vi "SetNag_report.vi"() -> ()   [LabVIEW 2013]
panel:
  out "Read 14":string
  in  "Write 13":string
  out "Read 13":string
  in  "Write 12":string
  out "Read 12":string
  in  "Write 11":string
  out "Read 11":string
  in  "Write 10":string
  in  "Write 9":string
  out "Read 10":string
  out "Read 9":string
  in  "Write 8":string
  in  "Write 7":string
  out "Read 8":string
  out "Read 7":string
  in  "Write 6":string
  out "Read 6":string
  in  "Write 5":string
  in  "milliseconds to wait":u32=250
  out "Read 5":string
  in  "Write 4":string
  out "Read 3":string
  in  "Baud Rate 2":i32(ring)=2 items=["2400", "4800", "9600", "19200", "38400", "57600", "115200"]
  in  "Com Port 2":i32(ring) items=["Com 1", "Com 2", "Com 3", "Com 4", "Com 5", "Com 6", "COM 7", "COM 8", "COM 9", "COM 10", "COM 11", "COM 12", "com 13", "COM 14"]
  in  "Write 3":string
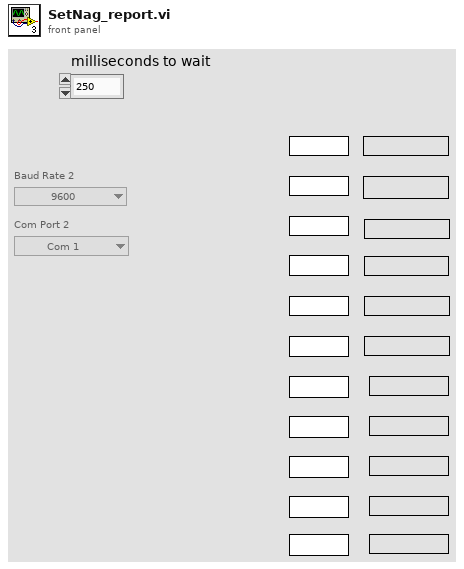
[diagram p1: front panel]
types:
  T1 = enum16{"no parity", "odd parity", "even parity", "mark parity", "space parity"}
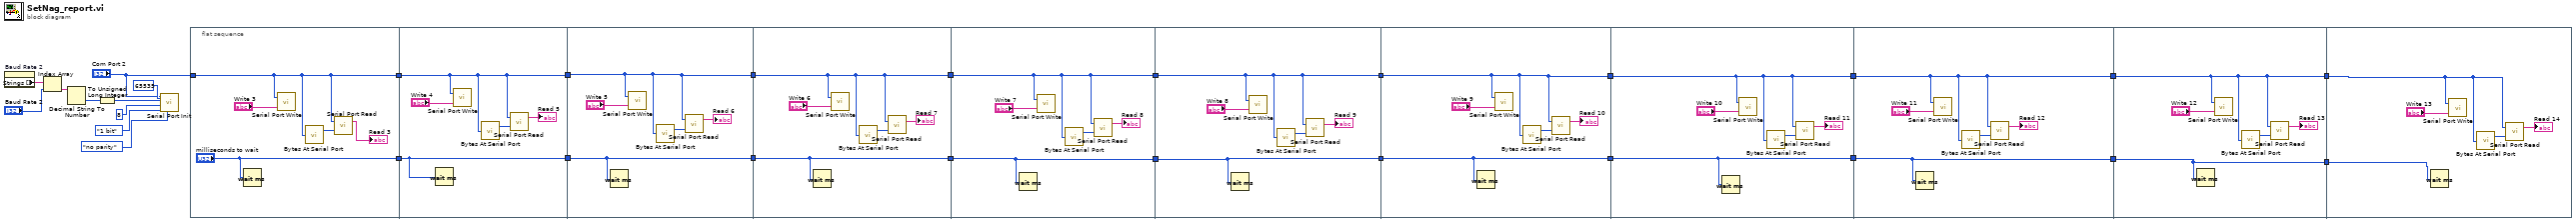
[diagram p0: block diagram]
diagram:
  n1 = property on="Baud Rate 2" class="Ring (strict)"() -> ("Strings []"=w23:string[])  [unwired: 2 in, 2 out]
  n2 = Index Array(array=w23, index="Baud Rate 2") -> (element=w24:string)
  n3 = Decimal String To Number(string=w24) -> (number=w22:i32)  [unwired: 2 in, 1 out]
  n4 = To Unsigned Long Integer(number=w22) -> (unsigned 32bit integer=w25:u32)
  n5 = call <vilib>:"Serial Port Init.vi"("parity"=T1."no parity", "buffer size"=u16 65535, "stop bits"=enum16{"1 bit", "1.5 bits", "2 bits"}."1 bit", "data bits"=u16 8, "baud rate"=w25, "port number"="Com Port 2") -> ()  [unwired: 1 in, 1 out]
  n6 = flat-sequence {
    tunnel: "Com Port 2" -> [w33]
    tunnel: [w33] -> w20
    tunnel: ["milliseconds to wait"] -> w19
    tunnel: w20 -> [w37]
    tunnel: w19 -> [w36]
    tunnel: [w37] -> w18
    tunnel: [w36] -> w16
    tunnel: w18 -> [w42]
    tunnel: [w42] -> w17
    tunnel: w16 -> [w41]
    tunnel: [w41] -> w15
    tunnel: w17 -> [w47]
    tunnel: w15 -> [w46]
    tunnel: [w47] -> w14
    tunnel: [w46] -> w13
    tunnel: w14 -> [w52]
    tunnel: w13 -> [w51]
    tunnel: [w52] -> w12
    tunnel: [w51] -> w11
    tunnel: w12 -> [w57]
    tunnel: w11 -> [w56]
    tunnel: [w57] -> w10
    tunnel: [w56] -> w9
    tunnel: w10 -> [w62]
    tunnel: w9 -> [w61]
    tunnel: [w62] -> w8
    tunnel: [w61] -> w7
    tunnel: w8 -> [w66]
    tunnel: w7 -> [w67]
    tunnel: [w67] -> w6
    tunnel: [w66] -> w5
    tunnel: w6 -> [w71]
    tunnel: w5 -> [w72]
    tunnel: [w72] -> w4
    tunnel: [w71] -> w3
    tunnel: w4 -> [w77]
    tunnel: w3 -> [w76]
    tunnel: [w77] -> w2
    tunnel: [w76] -> w1
    tunnel: w2 -> [w82]
    tunnel: w1 -> [w81]
    frame #0 {
      n7 = Wait (ms)(milliseconds to wait="milliseconds to wait") -> ()  [unwired: 1 out]
      n8 = call <vilib>:"Serial Port Write.vi"("string to write"="Write 3", "port number"=w33) -> ()  [unwired: 1 out]
      n9 = call <vilib>:"Bytes At Serial Port.vi"("port number"=w33) -> ("byte count"=w34:u32)  [unwired: 1 out]
      n10 = call <vilib>:"Serial Port Read.vi"("requested byte count"=w34, "port number"=w33) -> ("string read"=→"Read 3":string)  [unwired: 1 out]
    }
    frame #1 {
      n11 = Wait (ms)(milliseconds to wait=w36) -> ()  [unwired: 1 out]
      n12 = call <vilib>:"Serial Port Write.vi"("string to write"="Write 4", "port number"=w37) -> ()  [unwired: 1 out]
      n13 = call <vilib>:"Bytes At Serial Port.vi"("port number"=w37) -> ("byte count"=w40:u32)  [unwired: 1 out]
      n14 = call <vilib>:"Serial Port Read.vi"("requested byte count"=w40, "port number"=w37) -> ("string read"=→"Read 5":string)  [unwired: 1 out]
    }
    frame #2 {
      n15 = Wait (ms)(milliseconds to wait=w41) -> ()  [unwired: 1 out]
      n16 = call <vilib>:"Serial Port Write.vi"("string to write"="Write 5", "port number"=w42) -> ()  [unwired: 1 out]
      n17 = call <vilib>:"Bytes At Serial Port.vi"("port number"=w42) -> ("byte count"=w43:u32)  [unwired: 1 out]
      n18 = call <vilib>:"Serial Port Read.vi"("requested byte count"=w43, "port number"=w42) -> ("string read"=→"Read 6":string)  [unwired: 1 out]
    }
    frame #3 {
      n19 = Wait (ms)(milliseconds to wait=w46) -> ()  [unwired: 1 out]
      n20 = call <vilib>:"Serial Port Write.vi"("string to write"="Write 6", "port number"=w47) -> ()  [unwired: 1 out]
      n21 = call <vilib>:"Bytes At Serial Port.vi"("port number"=w47) -> ("byte count"=w50:u32)  [unwired: 1 out]
      n22 = call <vilib>:"Serial Port Read.vi"("requested byte count"=w50, "port number"=w47) -> ("string read"=→"Read 7":string)  [unwired: 1 out]
    }
    frame #4 {
      n23 = Wait (ms)(milliseconds to wait=w51) -> ()  [unwired: 1 out]
      n24 = call <vilib>:"Serial Port Write.vi"("string to write"="Write 7", "port number"=w52) -> ()  [unwired: 1 out]
      n25 = call <vilib>:"Bytes At Serial Port.vi"("port number"=w52) -> ("byte count"=w55:u32)  [unwired: 1 out]
      n26 = call <vilib>:"Serial Port Read.vi"("requested byte count"=w55, "port number"=w52) -> ("string read"=→"Read 8":string)  [unwired: 1 out]
    }
    frame #5 {
      n27 = Wait (ms)(milliseconds to wait=w56) -> ()  [unwired: 1 out]
      n28 = call <vilib>:"Serial Port Write.vi"("string to write"="Write 8", "port number"=w57) -> ()  [unwired: 1 out]
      n29 = call <vilib>:"Bytes At Serial Port.vi"("port number"=w57) -> ("byte count"=w58:u32)  [unwired: 1 out]
      n30 = call <vilib>:"Serial Port Read.vi"("requested byte count"=w58, "port number"=w57) -> ("string read"=→"Read 9":string)  [unwired: 1 out]
    }
    frame #6 {
      n31 = Wait (ms)(milliseconds to wait=w61) -> ()  [unwired: 1 out]
      n32 = call <vilib>:"Serial Port Write.vi"("string to write"="Write 9", "port number"=w62) -> ()  [unwired: 1 out]
      n33 = call <vilib>:"Bytes At Serial Port.vi"("port number"=w62) -> ("byte count"=w65:u32)  [unwired: 1 out]
      n34 = call <vilib>:"Serial Port Read.vi"("requested byte count"=w65, "port number"=w62) -> ("string read"=→"Read 10":string)  [unwired: 1 out]
    }
    frame #7 {
      n35 = Wait (ms)(milliseconds to wait=w67) -> ()  [unwired: 1 out]
      n36 = call <vilib>:"Serial Port Write.vi"("string to write"="Write 10", "port number"=w66) -> ()  [unwired: 1 out]
      n37 = call <vilib>:"Bytes At Serial Port.vi"("port number"=w66) -> ("byte count"=w68:u32)  [unwired: 1 out]
      n38 = call <vilib>:"Serial Port Read.vi"("requested byte count"=w68, "port number"=w66) -> ("string read"=→"Read 11":string)  [unwired: 1 out]
    }
    frame #8 {
      n39 = Wait (ms)(milliseconds to wait=w71) -> ()  [unwired: 1 out]
      n40 = call <vilib>:"Serial Port Write.vi"("string to write"="Write 11", "port number"=w72) -> ()  [unwired: 1 out]
      n41 = call <vilib>:"Bytes At Serial Port.vi"("port number"=w72) -> ("byte count"=w75:u32)  [unwired: 1 out]
      n42 = call <vilib>:"Serial Port Read.vi"("requested byte count"=w75, "port number"=w72) -> ("string read"=→"Read 12":string)  [unwired: 1 out]
    }
    frame #9 {
      n43 = Wait (ms)(milliseconds to wait=w76) -> ()  [unwired: 1 out]
      n44 = call <vilib>:"Serial Port Write.vi"("string to write"="Write 12", "port number"=w77) -> ()  [unwired: 1 out]
      n45 = call <vilib>:"Bytes At Serial Port.vi"("port number"=w77) -> ("byte count"=w78:u32)  [unwired: 1 out]
      n46 = call <vilib>:"Serial Port Read.vi"("requested byte count"=w78, "port number"=w77) -> ("string read"=→"Read 13":string)  [unwired: 1 out]
    }
    frame #10 {
      n47 = Wait (ms)(milliseconds to wait=w81) -> ()  [unwired: 1 out]
      n48 = call <vilib>:"Serial Port Write.vi"("string to write"="Write 13", "port number"=w82) -> ()  [unwired: 1 out]
      n49 = call <vilib>:"Bytes At Serial Port.vi"("port number"=w82) -> ("byte count"=w85:u32)  [unwired: 1 out]
      n50 = call <vilib>:"Serial Port Read.vi"("requested byte count"=w85, "port number"=w82) -> ("string read"=→"Read 14":string)  [unwired: 1 out]
    }
  }
